vi "Edit Experiment.vi"(5 "Experiment ID":i32, 6 "error in (no error)":errorcluster, 7 "Remarks":string, 8 "Name":string, 9 "Database.lvlib:Data Store.lvclass":refnum<class "Data Store.lvclass">) -> (0 "error out":errorcluster, 2 "Database.lvlib:Data Store.lvclass 2":refnum<class "Data Store.lvclass">)   [LabVIEW 2012, in "Database.lvlib" / "Data Store.lvclass"]
uses:
  Data Store.lvclass
  <vilib>/addons/database/Auxilliary.llb/DB Tools Parameter Info.ctl
  <vilib>/addons/database/Auxilliary.llb/DB Tools DataTypes.ctl
  <vilib>/addons/database/Auxilliary.llb/DB Tools Parameter Dir.ctl
  Data Store.lvclass/Data Store.ctl
  <vilib>/addons/database/Command.llb/Cmd Set Parameter Value (C).vi
  <vilib>/addons/database/Command.llb/Cmd Execute.vi
  <vilib>/addons/database/Recordset.llb/Rec Destroy - Command.vi
  <vilib>/addons/database/Command.llb/Cmd Delete.vi
  <vilib>/addons/database/NI_Database_API.lvlib
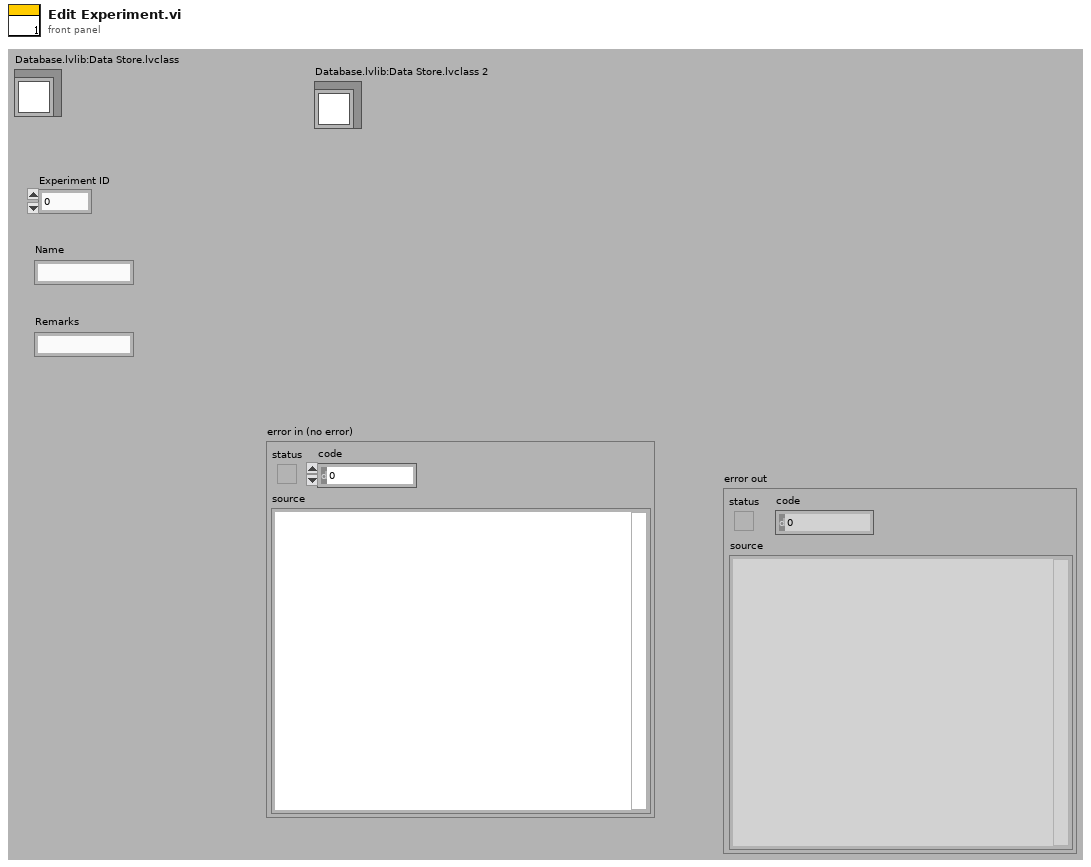
[diagram p1: front panel]
types:
  T1 = typedef "NI_Database_API.lvlib/DB Tools Parameter Info.ctl" = cluster{"parameter name":string, "type":T2, "direction":T3, "value":variant}
  T2 = typedef "NI_Database_API.lvlib/DB Tools DataTypes.ctl" = enum16{"String", "Long (I32)", "Single (SGL)", "Double (DBL)", "Date/Time", "Binary"}
  T3 = typedef "NI_Database_API.lvlib/DB Tools Parameter Dir.ctl" = enum32{"Input", "Output", "Input/Output", "Return Value"}
  T4 = typedef "NI_Database_API.lvlib/Conn ObjectReference.ctl" = refnum<k1>
  T5 = typedef "NI_Database_API.lvlib/Cmd ObjectReference.ctl" = refnum<k1>
  T6 = typedef "NI_Database_API.lvlib/Cmd-Rec Object Reference.ctl" = refnum<k1>
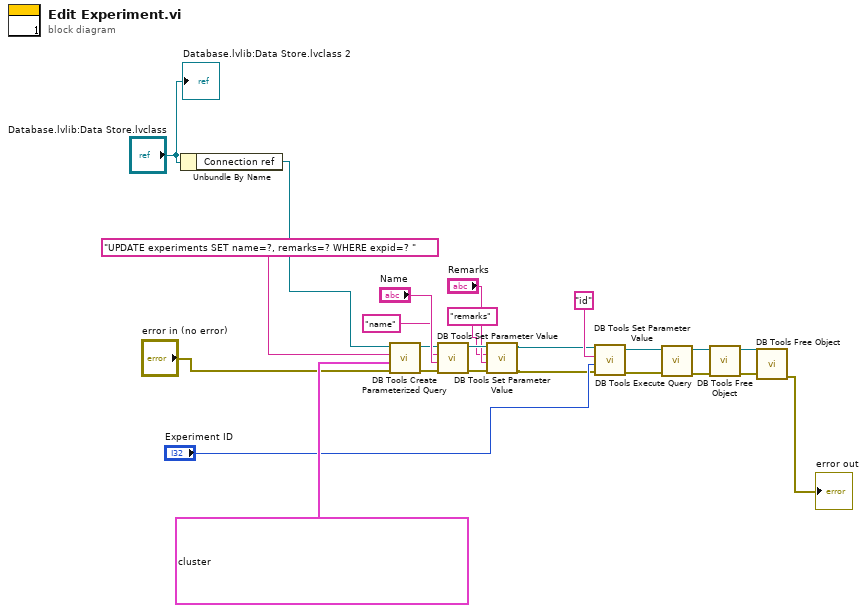
[diagram p0: block diagram]
diagram:
  n1 = Unbundle By Name("Database.lvlib:Data Store.lvclass") -> ("Connection ref"=w23:T4)
  n2 = call <vilib>:"DB Tools Create Parameterized Query.vi"("error in (no error)"="error in (no error)", "parameters"=T1[] [{"parameter name"="name", "type"=enum."String", "direction"=enum."Input", "value"=variant}, {"parameter name"="remarks", "type"=enum."String", "direction"=enum."Input", "value"=variant}, {"parameter name"="id", "type"=enum."Long (I32)", "direction"=enum."Input", "value"=variant}], "SQL query"="UPDATE experiments SET name=?, remarks=? WHERE expid=? ", "connection reference"=w23) -> ("error out"=w19:errorcluster, "command reference"=w15:T5)  [unwired: 3 in, 1 out]
  n3 = call-poly <vilib>:"DB Tools Set Parameter Value.vi"("error in (no error)"=w19, "value"="Name", "parameter index"="name", "command reference"=w15) -> ("error out"=w18:errorcluster, "command reference out"=w17:T5)  [unwired: 4 in]
  n4 = call-poly <vilib>:"DB Tools Set Parameter Value.vi"("error in (no error)"=w18, "value"="Remarks", "parameter index"="remarks", "command reference"=w17) -> ("error out"=w1:errorcluster, "command reference out"=w2:T5)  [unwired: 4 in]
  n5 = call-poly <vilib>:"DB Tools Set Parameter Value.vi"("error in (no error)"=w1, "value"="Experiment ID", "parameter index"="id", "command reference"=w2) -> ("error out"=w11:errorcluster, "command reference out"=w12:T5)  [unwired: 4 in]
  n6 = call-poly <vilib>:"DB Tools Execute Query.vi"("error in (no error)"=w11, "command reference"=w12) -> ("error out"=w10:errorcluster, "command-recordset reference"=w9:T6)  [unwired: 6 in]
  n7 = call-poly <vilib>:"DB Tools Free Object.vi"("error in (no error)"=w10, "command-recordset reference"=w9) -> ("error out"=w4:errorcluster, "command reference"=w5:T5)  [unwired: 8 in]
  n8 = call-poly <vilib>:"DB Tools Free Object.vi"("error in (no error)"=w4, "command reference"=w5) -> ("error out"=→"error out":errorcluster)  [unwired: 8 in, 1 out]
  "Database.lvlib:Data Store.lvclass 2" <- "Database.lvlib:Data Store.lvclass"
